vi "VISA Send Querry Recieve Message.vi"(0 "VISA session":refnum<visa-resource-name>, 7 "Send Message (\"\")":string="*IDN?", 9 "Timeout (25000)":u32=100, 11 "error in (no error)":errorcluster) -> (4 "dup VISA session":refnum<visa-resource-name>, 8 "Read Buffer":string, 15 "error out":errorcluster {"code" format="%.0x"})   [LabVIEW 2009]
doc: "This VI sends the message. Then it returns the response."
panel:
  in  "Command Termination":string="\n"
  in  "Read Temination":string="\n"
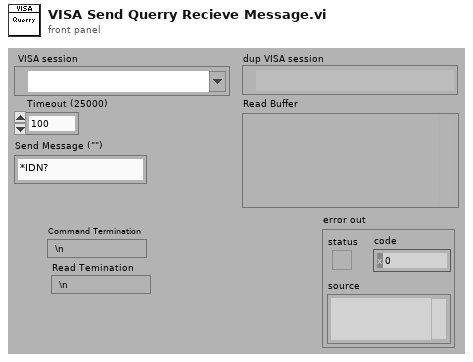
[diagram p1: front panel]
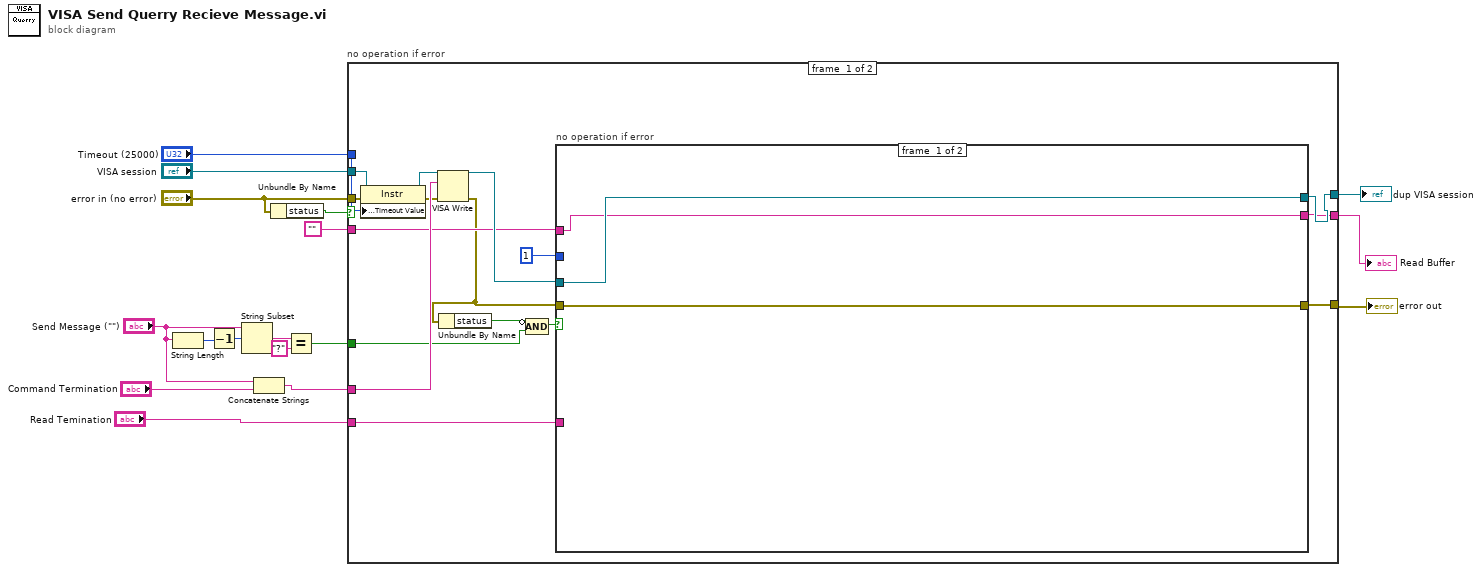
[diagram p0: block diagram]
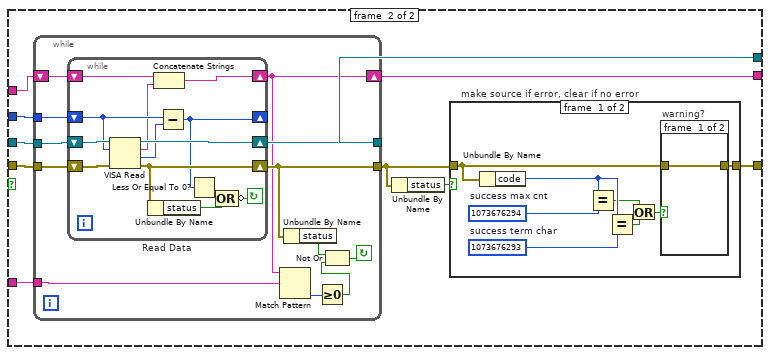
[diagram p2: hidden frame]
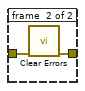
[diagram p3: hidden frame]
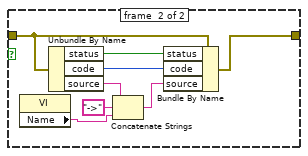
[diagram p4: hidden frame]
diagram:
  n1 = String Length(string="Send Message (\"\")") -> (length=w2:i32)
  n2 = Decrement(x=w2) -> (x-1=w1:i32)
  n3 = String Subset(string="Send Message (\"\")", offset (0)=w1) -> (substring=w5:string)  [unwired: 1 in]
  n4 = Concatenate Strings("Send Message (\"\")", "Command Termination") -> (w8:string)
  n5 = Unbundle By Name("error in (no error)") -> ("status"=w14:bool)
  n6 = Equal?(x=w5, y="?") -> (x = y?=w3:bool)
  n7 = case "no operation if error" shown="False" w14 {
    tunnel: "VISA session" -> [w31 w94]
    tunnel: w8 -> [w34 _]
    tunnel: [w25 w94] -> w13
    tunnel: [w27 w93] -> w17
    tunnel: "error in (no error)" -> [w33 w93]
    tunnel: "Timeout (25000)" -> [w29 _]
    tunnel: "" -> [w24 w92]
    tunnel: [w23 w92] -> w10
    tunnel: "Read Temination" -> [w22 _]
    tunnel: w3 -> [w18 _]
    frame #0 {
      n8 = property class="Instr"(reference=w31, error in=w33, "General Settings:Timeout Value"=w29) -> (reference out=w30:refnum<visa-resource-name>, error out=w32:errorcluster)
      n9 = VISA Write(VISA resource name=w30, write buffer=w34, error in (no error)=w32) -> (VISA resource name out=w26:refnum<visa-resource-name>, error out=w21:errorcluster)  [unwired: 1 out]
      n10 = Unbundle By Name(w21) -> ("status"=w19:bool)
      n11 = Compound Arithmetic op=AND(invert w19, w18) -> (w20:bool)
      n12 = case "no operation if error" shown="True" w20 {
        tunnel: [w36 w45] -> w25
        tunnel: [w37 w46] -> w27
        tunnel: u32 1 ("Byte (0)") -> [_ w47]
        tunnel: [w35 w39] -> w23
        tunnel: w21 -> [w37 w42]
        tunnel: w26 -> [w36 w41]
        tunnel: w24 -> [w35 w40]
        tunnel: w22 -> [_ w38]
        frame #0 {
        }
        frame #1 {
          n13 = while {
            tunnel: w47 -> [w59]
            tunnel: [w58] -> w45
            tunnel: [w53] -> w44
            tunnel: w42 -> [w57]
            tunnel: w41 -> [w56]
            shift-right: [w52] -> w39
            shift-left: w40 -> [w55]
            tunnel: w38 -> [w51]
            stop <- w48 continue-if-true
            n14 = while "Read Data" {
              shift-left: w55 -> [w67]
              shift-right: [w60] -> w52
              shift-left: w59 -> [w68]
              shift-right: [w63] -> _
              shift-left: w57 -> [w70]
              shift-right: [w65] -> w53
              shift-left: w56 -> [w72]
              shift-right: [w71] -> w58
              stop <- w61 continue-if-true
              n15 = VISA Read(VISA resource name=w72, byte count=w68, error in (no error)=w70) -> (VISA resource name out=w71:refnum<visa-resource-name>, read buffer=w66:string, return count=w69:u32, error out=w65:errorcluster)
              n16 = Unbundle By Name(w65) -> ("status"=w64:bool)
              n17 = Concatenate Strings(w67, w66) -> (w60:string)
              n18 = Subtract(x=w68, y=w69) -> (x-y=w63:u32)
              n19 = Less Or Equal To 0?(x=w63) -> (x <= 0?=w62:bool)
              n20 = Compound Arithmetic op=OR(w62, w64) -> (invert w61:bool)
            }
            n21 = Match Pattern(string=w52, regular expression=w51) -> (offset past match=w50:i32)  [unwired: 1 in, 3 out]
            n22 = Unbundle By Name(w53) -> ("status"=w54:bool)
            n23 = Greater Or Equal To 0?(x=w50) -> (x >= 0?=w49:bool)
            n24 = Not Or(1:w49, 2:w54) -> (0:w48:bool)
          }
          n25 = Unbundle By Name(w44) -> ("status"=w43:bool)
          n26 = case "make source if error, clear if no error" shown="False" w43 {
            tunnel: w44 -> [w74 w91]
            tunnel: [w73 w90] -> w46
            frame #0 {
              w79 = u32 1073676293  # success term char
              w80 = u32 1073676294  # success max cnt
              n27 = Unbundle By Name(w74) -> ("code"=w78:i32)
              n28 = Equal?(x=w78, y=w80) -> (x = y?=w77:bool)
              n29 = Equal?(x=w78, y=w79) -> (x = y?=w76:bool)
              n30 = Or(x=w77, y=w76) -> (x .or. y?=w75:bool)
              n31 = case "warning?" shown="True" w75 {
                tunnel: w74 -> [w81 w83]
                tunnel: [w81 w82] -> w73
                frame #0 {
                }
                frame #1 {
                  n32 = call <vilib>:"Clear Errors.vi"("error in (no error)"=w83) -> ("error out"=w82:errorcluster)  [unwired: 6 in]
                }
              }
            }
            frame #1 {
              n33 = property class="VI"() -> ("Name"=w84:string)  [unwired: 2 in, 2 out]
              n34 = Unbundle By Name(w91) -> ("status"=w89:bool, "code"=w88:i32, "source"=w87:string)
              n35 = Concatenate Strings(w87, "->", w84) -> (w86:string)
              n36 = Bundle By Name(cluster=w91, "status"=w89, "code"=w88, "source"=w86) -> (w90:errorcluster)
            }
          }
        }
      }
    }
    frame #1 {
    }
  }
  "error out" <- w17
  "dup VISA session" <- w13
  "Read Buffer" <- w10
